vi "svc_Unwrap Phase.vi"(6 "start phase":dbl, 10 "full cycle (2pi)":dbl=6.283185307179586 format="%.15f", 11 "phase in":dbl[](array[numeric])) -> (3 "phase out":dbl[](array[numeric]), 4 "end phase":dbl)   [LabVIEW 2017]
doc: "The phase array is unwrapped to remove discontinuities greater than pi. The start phase value is used as the start reference for the first element in the phase array."
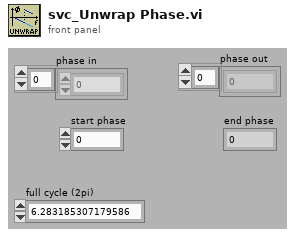
[diagram p1: front panel]
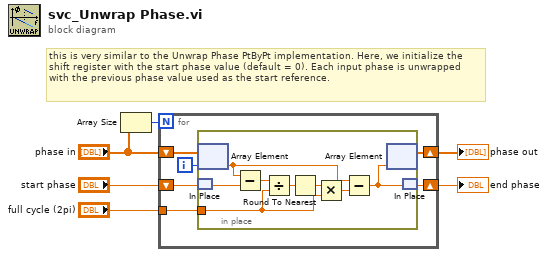
[diagram p0: block diagram]
diagram:
  # "this is very similar to the Unwrap Phase PtByPt implementation. Here, we initialize the shift register with the start phase value (default = 0). Each input phase is unwrapped with the previous phase value used as the start reference."
  n1 = Array Size(array="phase in") -> (size(s)=w2:i32)
  n2 = for {
    N: w2 -> [_]
    shift-right: [w7] -> w4
    shift-left: "start phase" -> [w9]
    tunnel: "full cycle (2pi)" -> [w12]
    shift-right: [w8] -> w5
    shift-left: "phase in" -> [w11]
    i -> [w10]
    n3 = in-place {
      in-place-border: w12 -> [w19]
      n4 = in-place-array #1(w11, w10) -> (w15:dbl)
      n5 = in-place-match #2(w9) -> (w14:dbl)
      n6 = Subtract(x=w15, y=w14) -> (x-y=w20:dbl)
      n7 = Divide(x=w20, y=w19) -> (x/y=w18:dbl)
      n8 = Round To Nearest(number=w18) -> (nearest integer value=w16:dbl)
      n9 = Multiply(x=w16, y=w19) -> (x*y=w17:dbl)
      n10 = Subtract(x=w15, y=w17) -> (x-y=w13:dbl)
      n11 = in-place-array #1(w13) -> (w8:dbl[])  [unwired: 1 out]
      n12 = in-place-match #2(w13) -> (w7:dbl)
    }
  }
  "phase out" <- w5
  "end phase" <- w4
